vi "Make_Settings_Item.vi"(8 "error in (no error)":errorcluster, 10 "address":string[](array[string]), 11 "IB_Source in":refnum<class "IB_Source.lvclass">) -> (0 "error out":errorcluster, 3 "IB_Settings_Item.lvclass":refnum<class "IB_Settings_Item.lvclass">)   [LabVIEW 2020, in "IB_Source.lvclass"]
uses:
  <vilib>/AppBuilder/IB_Classes/Source/IB_Source.lvclass
  <vilib>/AppBuilder/IB_Classes/Source/IB_Source.lvclass/IB_Source.ctl
  <vilib>/AppBuilder/IB_Classes/Settings_Item/IB_Settings_Item.lvclass
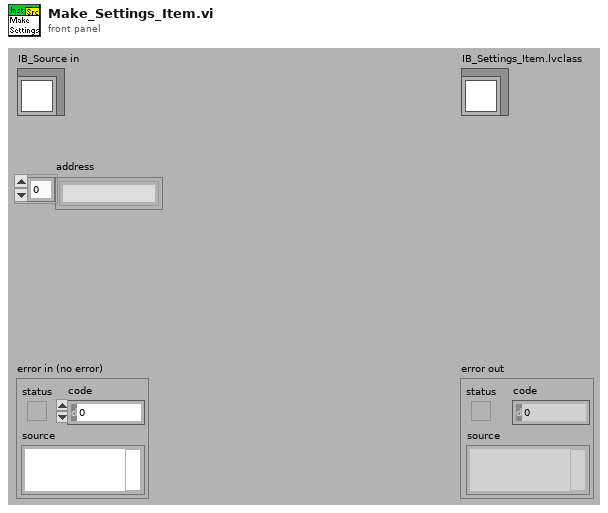
[diagram p1: front panel]
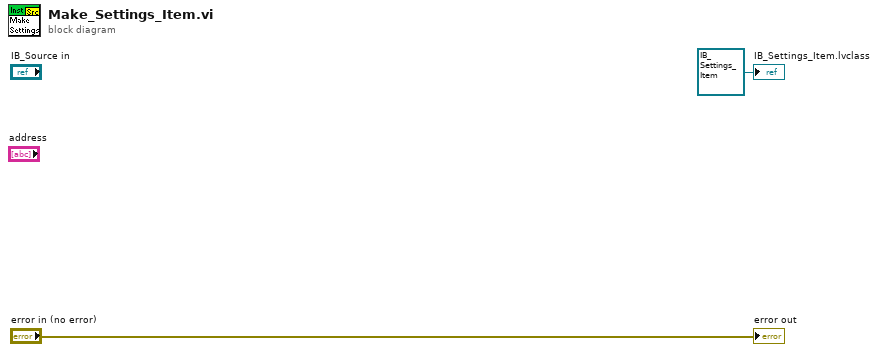
[diagram p0: block diagram]
diagram:
  "error out" <- "error in (no error)"
  "IB_Settings_Item.lvclass" <- refnum<class "IB_Settings_Item.lvclass"> refnum ("IB_Settings_Item.lvclass")
